vi "Telnet Write.vi"(4 "line separator (\\n)":string="\n", 5 "write mode (normal)":enum16{"normal", "line", "buffered"}(ring), 6 "error in (no error)":errorcluster, 7 "timeout ms (25000)":i32=25000, 8 "data in":string, 9 "telnet connection":T1) -> (0 "error out":errorcluster, 1 "bytes written":i32, 3 "telnet  connection out":T1)   [LabVIEW 2015]
doc: "Writes data to a connection opened with Telnet Open Connection, escapping special characters.\n\nwrite mode:\n normal (same as TCP Write)\n line (replaces EOLN characters with the line separator and writes the entire buffer ignoring the timout)\n buffered (writes the entire buffer ignoring the timeout)"
uses:
  Telnet Session.ctl
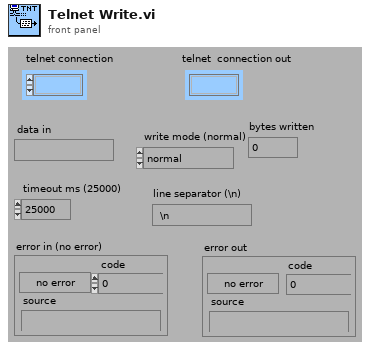
[diagram p1: front panel]
types:
  T1 = typedef "Telnet Session.ctl" = refnum<k1>
  T2 = typedef "Telnet Connection Data.ctl" = cluster{"id":refnum<k5>, "read sem":T3, "write sem":T3, "read buffer":string, "read unfiltered buffer":string}
  T3 = typedef "Semaphore RefNum.ctl" = refnum<k1>
  T4 = cluster{"timeout ms (25000)":i32, "timeout ms (25000)":i32, "write mode (normal)":enum16{"normal", "line", "buffered"}, "line separator (\\n)":string}
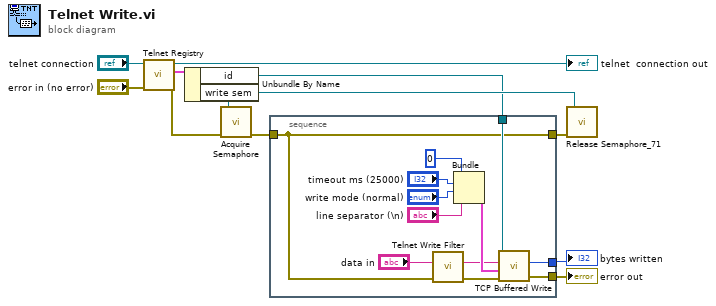
[diagram p0: block diagram]
diagram:
  n1 = call "Telnet Registry.vi"("error in (no error)"="error in (no error)", "object"="telnet connection") -> ("error out"=w4:errorcluster, "object data"=w6:T2, "object out"=→"telnet  connection out":T1)  [unwired: 5 in, 2 out]
  n2 = Unbundle By Name(w6) -> ("id"=w5:refnum<k5>, "write sem"=w7:T3)
  n3 = call <vilib>:"Acquire Semaphore.vi"("error in (no error)"=w4, "semaphore"=w7) -> ("error out"=w2:errorcluster)  [unwired: 3 in, 2 out]
  n4 = stacked-sequence {
    tunnel: w5 -> [w22]
    tunnel: [w21] -> w10
    tunnel: [w15] -> w11
    tunnel: w2 -> [w14]
    tunnel: [w14] -> w1
    frame #0 {
      n5 = call "Telnet Write Filter.vi"("Data"="data in") -> ("Data out"=w12:string)
      n6 = Bundle("timeout ms (25000)"=0, "timeout ms (25000)"="timeout ms (25000)", "write mode (normal)"="write mode (normal)", "line separator (\\n)"="line separator (\\n)") -> (w20:T4)  [unwired: 1 in]
      n7 = call "TCP Buffered Write.vi"("error in (no error)"=w14, "read/write info"=w20, "data in"=w12, "connection ID"=w22) -> ("error out"=w21:errorcluster, "bytes written"=w15:i32)  [unwired: 5 in, 1 out]
    }
  }
  "bytes written" <- w11
  "error out" <- w10
  n8 = call <vilib>:"Release Semaphore_71.vi"("error in (no error)"=w1, "semaphore"=w7) -> ()  [unwired: 4 in, 2 out]
